vi "QA-Trace Error.vi"(7 "trace integer":i32, 11 "error in (no error)":errorcluster) -> (15 "error out":errorcluster)   [LabVIEW 2015]
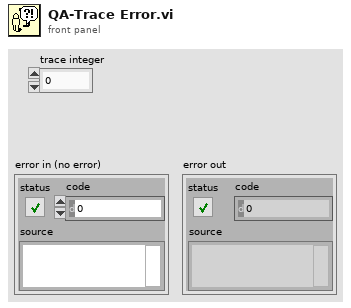
[diagram p1: front panel]
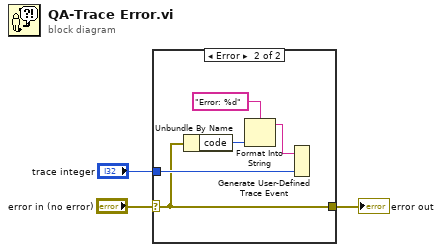
[diagram p0: block diagram]
diagram:
  n1 = case shown="Error" "error in (no error)" {
    selector: "error in (no error)" -> [w4 w8]
    tunnel: "trace integer" -> [_ w9]
    tunnel: [w4 w8] -> w1
    frame No Error {
    }
    frame Error {
      n2 = Unbundle By Name(w8) -> ("code"=w5:i32)
      n3 = Format Into String(format string="Error: %d", w5) -> (resulting string=w7:string)  [unwired: 2 in, 1 out]
      n4 = Generate User-Defined Trace Event(1:w9, 2:w7) -> ()
    }
  }
  "error out" <- w1
